vi "json_parse.vi"() -> (1 "SpecCurrent":dbl, 2 "ScanCurrent":dbl, 3 "Path":path)   [LabVIEW 2019]
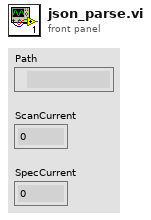
[diagram p1: front panel]
types:
  T1 = cluster{"Nanonis_Settings":cluster{"ScanCurrent":dbl, "SpecCurrent":dbl, "FolderLocation":string}}
  T2 = cluster{"ScanCurrent":dbl, "SpecCurrent":dbl, "FolderLocation":string}
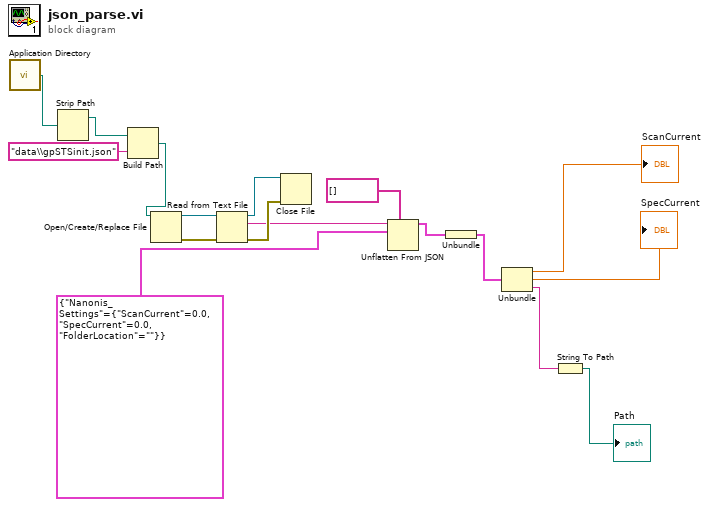
[diagram p0: block diagram]
diagram:
  n1 = call <vilib>:"Application Directory.vi"() -> ("Application Directory"=w11:path)
  n2 = Strip Path(path=w11) -> (stripped path=w3:path)  [unwired: 1 out]
  n3 = Build Path(base path=w3, name or relative path="data\\gpSTSinit.json") -> (appended path=w1:path)
  n4 = Open/Create/Replace File(file path (use dialog)=w1) -> (refnum out=w9:refnum<file>, error out=w10:errorcluster)  [unwired: 5 in, 1 out]
  n5 = Read from Text File(file (use dialog)=w9, error in=w10) -> (refnum out=w8:refnum<file>, text=w6:string, error out=w7:errorcluster)  [unwired: 2 in, 1 out]
  n6 = Close File(refnum=w8, error in=w7) -> ()  [unwired: 2 out]
  n7 = Unflatten From JSON(path=string[] [], JSON string=w6, type and defaults=T1 {"Nanonis_Settings"={"ScanCurrent"=0.0, "SpecCurrent"=0.0, "FolderLocation"=""}}) -> (value=w12:T1)  [unwired: 4 in, 1 out]
  n8 = Unbundle(w12) -> ("Nanonis_Settings"=w13:T2)
  n9 = Unbundle(w13) -> ("ScanCurrent"=→"ScanCurrent":dbl, "SpecCurrent"=→"SpecCurrent":dbl, "FolderLocation"=w16:string)
  n10 = String To Path(string=w16) -> (path=→"Path":path)
